vi "Test To Report Entry.vi"(8 "error in (no error)":errorcluster, 10 "Test Node":T1) -> (0 "error out":errorcluster, 2 "String":string)   [LabVIEW 2020, in "Caraya.lvlib" / "Test Report.Template.lvclass"]
uses:
  Test Report.Template.lvclass
  Test Result/Test Node (Extended).ctl
  Test Result/Test Registration Data.ctl
  Test Report/Test Report.lvclass
  Test Result/Test Result.lvclass
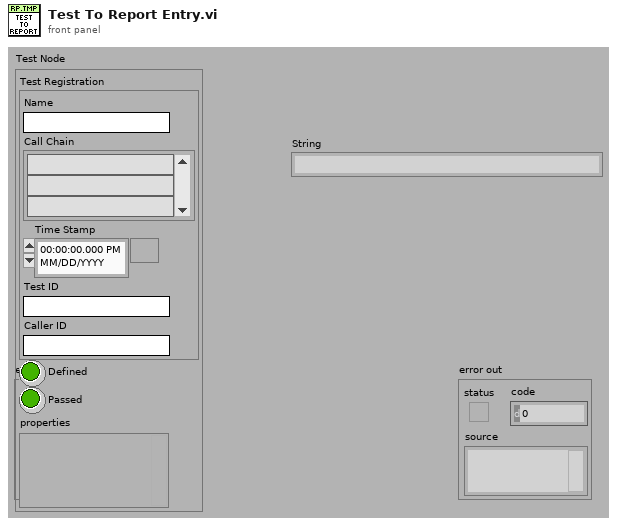
[diagram p1: front panel]
types:
  T1 = typedef "Caraya.lvlib/Test Result.lvclass/Test Node (Extended).ctl" = cluster{"Test Registration":T2, "Defined":bool, "Passed":bool, "properties":variant}
  T2 = typedef "Caraya.lvlib/Test Result.lvclass/Test Registration Data.ctl" = cluster{"Name":string, "Call Chain":string[], "Time Stamp":timestamp, "Test ID":string, "Caller ID":string}
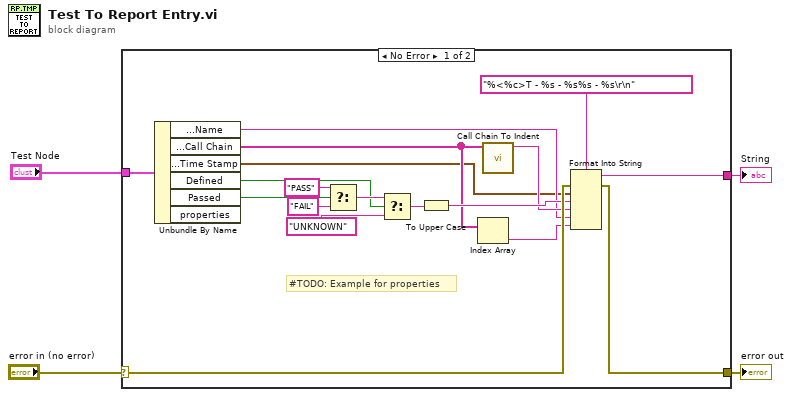
[diagram p0: block diagram]
diagram:
  n1 = case shown="No Error" "error in (no error)" {
    selector: "error in (no error)" -> [w20 w23]
    tunnel: [w19 w23] -> w3
    tunnel: "Test Node" -> [w22 _]
    tunnel: [w13 _] -> w1
    frame No Error {
      # "#TODO: Example for properties"
      n2 = Unbundle By Name(w22) -> ("Test Registration.Name"=w15:string, "Test Registration.Call Chain"=w16:string[], "Test Registration.Time Stamp"=w12:timestamp, "Defined"=w7:bool, "Passed"=w9:bool)  [unwired: 1 out]
      n3 = Select(t="PASS" ("format string"), s=w9, f="FAIL" ("format string")) -> (s? t:f=w11:string)
      n4 = Select(t=w11, s=w7, f="UNKNOWN" ("format string")) -> (s? t:f=w5:string)
      n5 = To Upper Case(1:w5) -> (0:w18:string)
      n6 = Index Array(array=w16) -> (element=w14:string)  [unwired: 1 in]
      n7 = call "Call Chain To Indent.vi"("Call Chain"=w16) -> ("Indent"=w17:string)  [unwired: 10 in]
      n8 = Format Into String(format string="%<%c>T - %s - %s%s - %s\r\n", error in=w20, w12, w18, w17, w15, w14) -> (resulting string=w13:string, error out=w19:errorcluster)  [unwired: 1 in]
    }
    frame Error {
    }
  }
  "error out" <- w3
  "String" <- w1
